vi "rethinkdb_example_cursor.vi"() -> ()   [LabVIEW 2017]
uses:
  rethinkdb/rethinkdb.lvlib
  rethinkdb/run_cursor.vi
panel:
  out "object count":i32
  out "object":variant
  out "debug":string
  out "error out":errorcluster
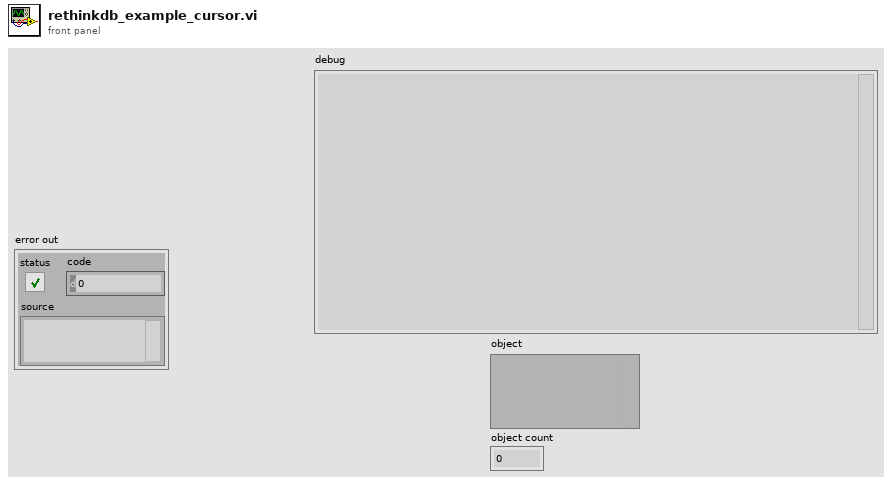
[diagram p1: front panel]
types:
  T1 = typedef "rethinkdb.lvlib/refnum.ctl" = refnum<k1>
  T2 = typedef "rethinkdb.lvlib/cursor_refnum.ctl" = refnum<k1>
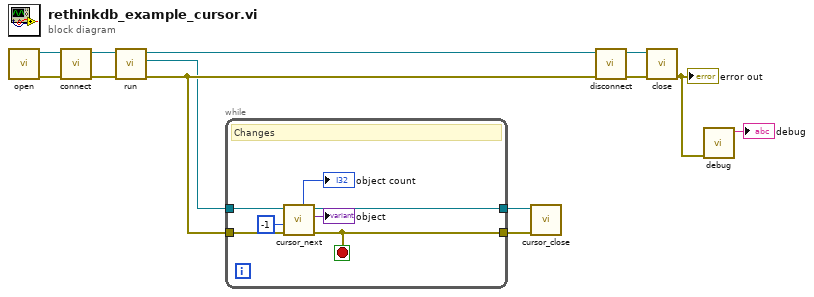
[diagram p0: block diagram]
diagram:
  n1 = call "open.vi"() -> ("error out"=w13:errorcluster, "rethinkdb"=w12:T1)  [unwired: 10 in]
  n2 = call "connect.vi"("error in (no error)"=w13, "rethinkdb in"=w12) -> ("error out"=w7:errorcluster, "rethinkdb out"=w6:T1)  [unwired: 8 in]
  n3 = call-poly "run.vi"("error in (no error)"=w7, "rethinkdb in"=w6) -> ("error out"=w4:errorcluster, "cursor"=w3:T2, "rethinkdb out"=w5:T1)  [unwired: 7 in]
  n4 = while {
    tunnel: w4 -> [w20]
    tunnel: w3 -> [w19]
    tunnel: [w15] -> w2
    tunnel: [w14] -> w1
    stop <- w14 stop-if-true
    # "Changes"
    n5 = call "cursor_next.vi"("error in (no error)"=w20, "ms wait (-1)"=-1, "cursor in"=w19) -> ("error out"=w14:errorcluster, "object"=→"object":variant, "cursor out"=w15:T2, "object count"=→"object count":i32)  [unwired: 4 in, 1 out]
  }
  n6 = call "cursor_close.vi"("error in (no error)"=w1, "cursor"=w2) -> ()  [unwired: 9 in, 1 out]
  n7 = call "disconnect.vi"("error in (no error)"=w4, "rethinkdb in"=w5) -> ("error out"=w11:errorcluster, "rethinkdb out"=w10:T1)  [unwired: 8 in]
  n8 = call "close.vi"("error in (no error)"=w11, "rethinkdb"=w10) -> ("error out"=w9:errorcluster)  [unwired: 9 in]
  "error out" <- w9
  n9 = call "debug.vi"("error in (no error)"=w9) -> ("debug"=→"debug":string)  [unwired: 9 in, 1 out]
